vi "PiezoCloseSynchronization.vi"(7 "PiezoSynchronization":T1, 9 "error in (no error)":errorcluster) -> (6 "error out":errorcluster)   [LabVIEW 2009]
uses:
  Controls/PiezoSynchronization.ctl
  Controls/PIEZO.COMMAND.QUEUE.ctl
  Controls/PIEZO.COMMAND.ctl
  Controls/PIEZO.COMMANDBASIC.ctl
  Controls/PIEZO.WAVE.ctl
  Controls/PIEZO.STATE.ctl
  Controls/PIEZO.WAVE.NOTIFIER.ctl
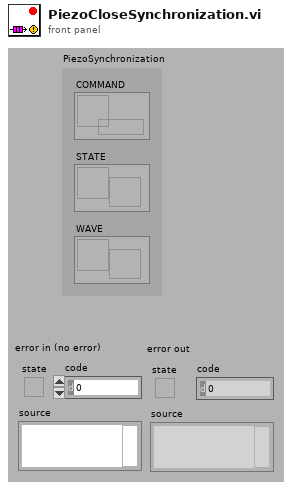
[diagram p1: front panel]
types:
  T1 = typedef "PiezoSynchronization.ctl" = cluster{"COMMAND":T2, "STATE":refnum<notifier>, "WAVE":T3}
  T2 = typedef "PIEZO.COMMAND.QUEUE.ctl" = refnum<queue>
  T3 = typedef "PIEZO.WAVE.NOTIFIER.ctl" = refnum<notifier>
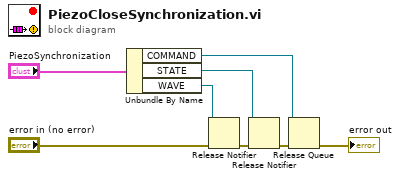
[diagram p0: block diagram]
diagram:
  n1 = Unbundle By Name("PiezoSynchronization") -> ("COMMAND"=w1:T2, "STATE"=w2:refnum<notifier>, "WAVE"=w3:T3)
  n2 = Release Notifier(notifier=w3, error in (no error)="error in (no error)") -> (error out=w6:errorcluster)  [unwired: 1 in, 2 out]
  n3 = Release Notifier(notifier=w2, error in (no error)=w6) -> (error out=w5:errorcluster)  [unwired: 1 in, 2 out]
  n4 = Release Queue(queue=w1, error in (no error)=w5) -> (error out=→"error out":errorcluster)  [unwired: 1 in, 2 out]
